vi "Count.vi"(8 "错误输入":errorcluster, 11 "Mlistbox Ref":refnum<vi>) -> (0 "错误输出":errorcluster, 2 "Count":i32, 3 "Mlistbox Ref Dup":refnum<vi>)   [LabVIEW 2012, in "Mlistbox Tools.lvlib"]
uses:
  Mlistbox Tools.lvlib
  ListBox/Custom Type/Read and Write Mode.ctl
  Property/Set and Get ItemNames.vi
  ListBox/Listbox Tool.lvlib
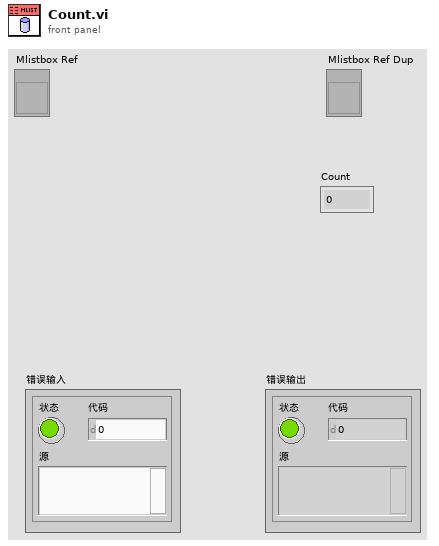
[diagram p1: front panel]
types:
  T1 = typedef "Listbox Tool.lvlib/Read and Write Mode.ctl" = enum16{"Read", "Write"}
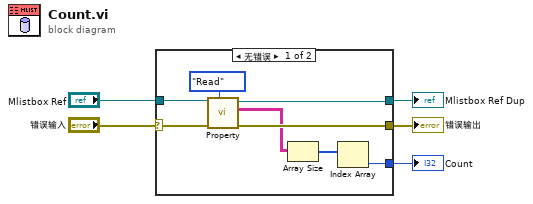
[diagram p0: block diagram]
diagram:
  n1 = case shown="无错误" "错误输入" {
    selector: "错误输入" -> [w11 w15]
    tunnel: [w9 w15] -> w4
    tunnel: "Mlistbox Ref" -> [w13 w14]
    tunnel: [w10 w14] -> w2
    tunnel: [w6 _] -> w1
    frame No Error {
      n2 = call-poly "Property.vi"("Mode"=Read_and_Write_Mode."Read", "错误输入"=w11, "Mlistbox Ref"=w13) -> ("错误输出"=w9:errorcluster, "ItemNames Out"=w8:string[][], "Mlistbox Ref Dup"=w10:refnum<vi>)  [unwired: 6 in]
      n3 = Array Size(array=w8) -> (size(s)=w7:i32[])
      n4 = Index Array(array=w7) -> (element=w6:i32)  [unwired: 1 in]
    }
    frame Error {
    }
  }
  "Mlistbox Ref Dup" <- w2
  "错误输出" <- w4
  "Count" <- w1
